vi "Edit Custom Device Project.vi"() -> ()   [LabVIEW 2010]
panel:
  in  "Template Files Folder":path
  in  "Custom Device Folder":path
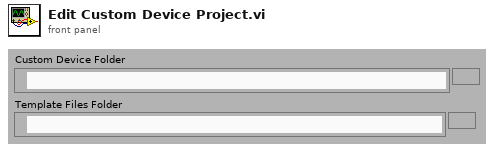
[diagram p1: front panel]
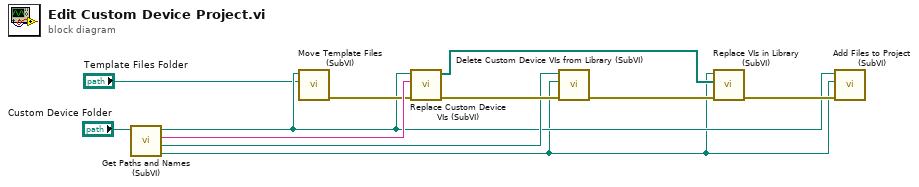
[diagram p0: block diagram]
diagram:
  n1 = call "Get Paths and Names (SubVI).vi"("Custom Device Folder"="Custom Device Folder") -> ("Custom Device Library"=w2:path, "Custom Device Project"=w4:path, "Custom Device Name"=w10:string, "Custom Device Folder"=w3:path)  [unwired: 7 in]
  n2 = call "Move Template Files (SubVI).vi"("Template Files Path"="Template Files Folder", "Custom Device Folder"=w3) -> ("error out"=w8:errorcluster)  [unwired: 9 in]
  n3 = call "Replace Custom Device VIs (SubVI).vi"("error out"=w8, "Custom Device Name"=w10, "Custom Device Folder"=w3) -> ("error out 2"=w7:errorcluster, "Custom Device VIs"=w9:path[])  [unwired: 7 in]
  n4 = call "Delete Custom Device VIs from Library (SubVI).vi"("error out 2"=w7, "Custom Device Library"=w2, "Custom Device Project"=w4) -> ("error out"=w6:errorcluster)  [unwired: 8 in]
  n5 = call "Replace VIs in Library (SubVI).vi"("error out"=w6, "Custom Device VIs"=w9, "Custom Device Library"=w2) -> ("error out 2"=w5:errorcluster)  [unwired: 8 in]
  n6 = call "Add Files to Project (SubVI).vi"("error out 2"=w5, "Custom Device Library"=w2, "Custom Device Folder"=w3) -> ()  [unwired: 9 in]
